vi "Get Relay Status Array.vi"(8 "error in (no error)":errorcluster, 11 "SLSC Switch in":refnum<class "SLSC Switch.lvclass">) -> (0 "error out":errorcluster, 1 "Closed Relays":string[](array[string]), 2 "Relay Status Array":T1[](array[typedef]), 3 "SLSC Switch out":refnum<class "SLSC Switch.lvclass">)   [LabVIEW 2016, in "SLSC Switch.lvlib" / "SLSC Switch.lvclass"]
uses:
  SLSC Switch.lvclass
  Controls/Relay Status.ctl
  Relay/Relay Position.ctl
  SLSC Switch.lvclass/SLSC Switch.ctl
  Relay/Relay.lvclass/Relay.ctl
  Switch Action Processor/Switch Action Processor.lvclass
  Relay/Relay.lvclass
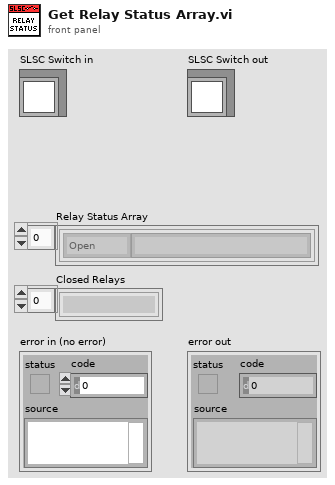
[diagram p1: front panel]
types:
  T1 = typedef "SLSC Switch.lvlib/SLSC Switch.lvclass/Relay Status.ctl" = cluster{"position":T2, "Name":string}
  T2 = typedef "SLSC Switch.lvlib/Relay.lvclass/Relay Position.ctl" = enum16{"Open", "Closed"}
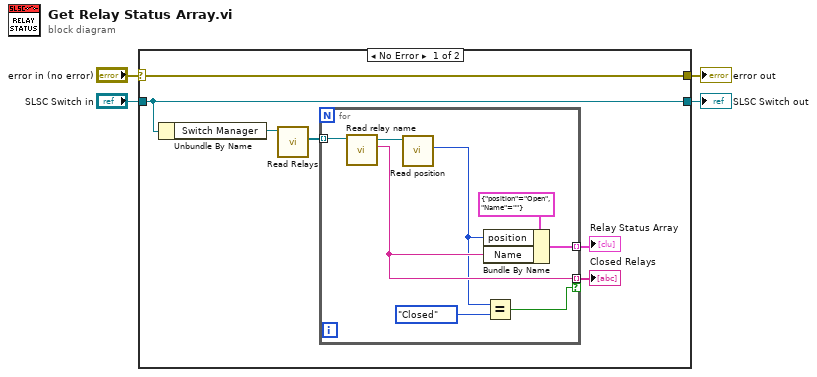
[diagram p0: block diagram]
diagram:
  n1 = case shown="No Error" "error in (no error)" {
    selector: "error in (no error)" -> [w10 w20]
    tunnel: [w10 w20] -> w3
    tunnel: "SLSC Switch in" -> [w9 w19]
    tunnel: [w9 w19] -> w1
    frame No Error {
      n2 = Unbundle By Name(w9) -> ("Switch Manager"=w8:refnum<class "Switch Action Processor.lvclass">)
      n3 = call-dynamic "Read Relays.vi"("Switch Action Processor in"=w8) -> ("Relays"=w7:refnum<class "Relay.lvclass">[])  [unwired: 8 in, 2 out]
      n4 = for {
        tunnel: w7 -> [w18] mode=indexing
        tunnel: [w15] -> w5 mode=indexing
        tunnel: [w14] -> w6 mode=indexing if=w11
        n5 = call "Read relay name.vi"("Relay in"=w18) -> ("name"=w14:string, "Relay out"=w17:refnum<class "Relay.lvclass">)  [unwired: 8 in, 1 out]
        n6 = call "Read position.vi"("Relay in"=w17) -> ("position"=w13:T2)  [unwired: 8 in, 2 out]
        n7 = Bundle By Name(cluster=T1 {"position"=enum."Open", "Name"=""} ("Relay Status"), "position"=w13, "Name"=w14) -> (w15:T1)
        n8 = Equal?(x=w13, y=Relay_Position."Closed") -> (x = y?=w11:bool)
      }
      "Closed Relays" <- w6
      "Relay Status Array" <- w5
    }
    frame Error {
    }
  }
  "error out" <- w3
  "SLSC Switch out" <- w1
